vi "Telescope Update Status.vi"(8 "error in":errorcluster, 10 "Telescope Status":T2, 11 "HK Channel in":refnum<class "HK Table.lvclass">) -> (0 "error out":errorcluster, 2 "alarms":T1[](array[typedef]), 3 "HK Channel out":refnum<class "HK Table.lvclass">)   [LabVIEW 2021, in "Telescope.lvclass"]
uses:
  Telescope.lvclass
  Telescope cluster Status.ctl
  typedefs/CC cluster RA and DEC.ctl
  Telescope enum Status.ctl
  hk-channel-class/HK Table/HK Table.lvclass
  hk-channel-class/HK Alarms/HK Alarm enum Status.ctl
  hk-channel-class/HK Item/HK Item.lvclass
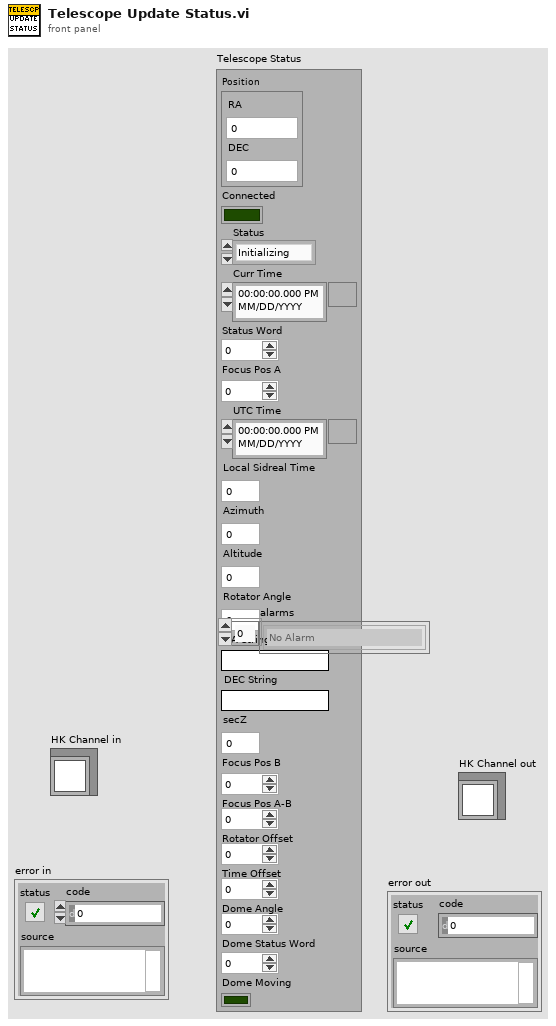
[diagram p1: front panel]
types:
  T1 = typedef "HK Item.lvclass/HK Alarm enum Status.ctl" = enum16{"No Alarm", "Red Low", "Red High", "Yellow Low", "Yellow High"}
  T2 = typedef "Telescope.lvclass/Telescope cluster Status.ctl" = cluster{"Position":T3, "Connected":bool, "Status":T4, "Curr Time":timestamp, "Status Word":u32, "Focus Pos A":dbl, "UTC Time":timestamp, "Local Sidreal Time":dbl, "Azimuth":dbl, "Altitude":dbl, "Rotator Angle":dbl, "RA String":string, "DEC String":string, "secZ":dbl, "Focus Pos B":dbl, "Focus Pos A-B":dbl, "Rotator Offset":dbl, "Time Offset":dbl, "Dome Angle":dbl, "Dome Status Word":u32, "Dome Moving":bool}
  T3 = typedef "CC cluster RA and DEC.ctl" = cluster{"RA":dbl, "DEC":dbl}
  T4 = typedef "Telescope.lvclass/Telescope enum Status.ctl" = enum16{"Initializing", "Ready", "Moving", "Focusing", "Error"}
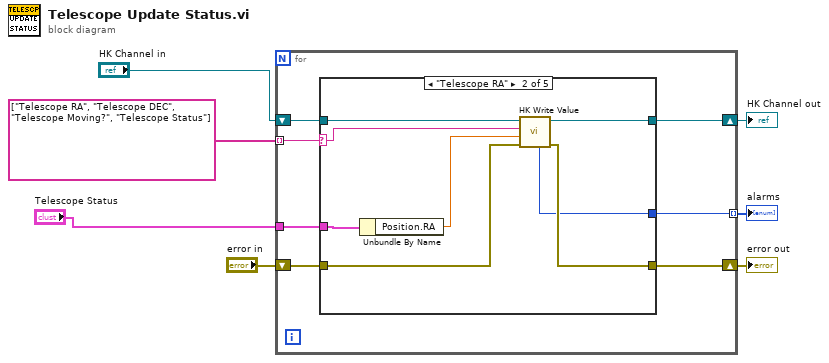
[diagram p0: block diagram]
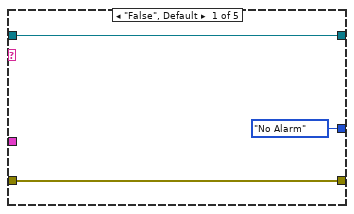
[diagram p2: hidden frame]
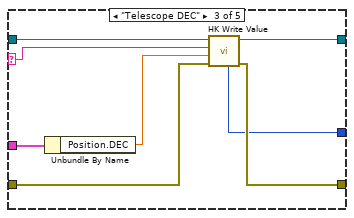
[diagram p3: hidden frame]
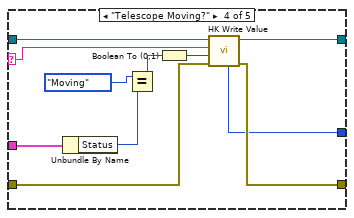
[diagram p4: hidden frame]
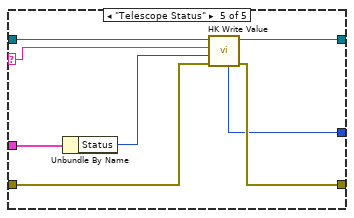
[diagram p5: hidden frame]
diagram:
  n1 = for {
    tunnel: string[] ["Telescope RA", "Telescope DEC", "Telescope Moving?", "Telescope Status"] -> [w14] mode=indexing
    shift-right: [w13] -> w2
    shift-left: "HK Channel in" -> [w12]
    shift-right: [w10] -> w4
    shift-left: "error in" -> [w11]
    tunnel: "Telescope Status" -> [w9]
    tunnel: [w8] -> w1 mode=indexing
    n2 = case shown="\"Telescope RA\"" w14 {
      selector: w14 -> [_ w23 w31 w42 w50]
      tunnel: [w17 w25 w33 w44 w52] -> w13
      tunnel: w12 -> [w17 w24 w32 w43 w51]
      tunnel: w11 -> [w16 w22 w30 w41 w49]
      tunnel: [w16 w21 w29 w40 w48] -> w10
      tunnel: w9 -> [_ w20 w28 w39 w47]
      tunnel: [HK_Alarm_enum_Status."No Alarm" ("Alarm Status") w18 w26 w34 w45] -> w8
      frame "False", Default {
      }
      frame "Telescope RA" {
        n3 = Unbundle By Name(w20) -> ("Position.RA"=w19:dbl)
        n4 = call-dynamic "HK Write Value.vi"("error in (no error)"=w22, "Value"=w19, "Channel Name"=w23, "HK Channel in"=w24) -> ("error out"=w21:errorcluster, "HK Channel out"=w25:refnum<class "HK Table.lvclass">, "Alarm Status"=w18:T1)  [unwired: 3 in, 2 out]
      }
      frame "Telescope DEC" {
        n5 = Unbundle By Name(w28) -> ("Position.DEC"=w27:dbl)
        n6 = call-dynamic "HK Write Value.vi"("error in (no error)"=w30, "Value"=w27, "Channel Name"=w31, "HK Channel in"=w32) -> ("error out"=w29:errorcluster, "HK Channel out"=w33:refnum<class "HK Table.lvclass">, "Alarm Status"=w26:T1)  [unwired: 3 in, 2 out]
      }
      frame "Telescope Moving?" {
        n7 = Unbundle By Name(w39) -> ("Status"=w38:T4)
        n8 = Equal?(x=Telescope_enum_Status."Moving" ("Status"), y=w38) -> (x = y?=w37:bool)
        n9 = Boolean To (0,1)(Boolean=w37) -> (0, 1=w35:i16)
        n10 = call-dynamic "HK Write Value.vi"("error in (no error)"=w41, "Value"=w35, "Channel Name"=w42, "HK Channel in"=w43) -> ("error out"=w40:errorcluster, "HK Channel out"=w44:refnum<class "HK Table.lvclass">, "Alarm Status"=w34:T1)  [unwired: 3 in, 2 out]
      }
      frame "Telescope Status" {
        n11 = Unbundle By Name(w47) -> ("Status"=w46:T4)
        n12 = call-dynamic "HK Write Value.vi"("error in (no error)"=w49, "Value"=w46, "Channel Name"=w50, "HK Channel in"=w51) -> ("error out"=w48:errorcluster, "HK Channel out"=w52:refnum<class "HK Table.lvclass">, "Alarm Status"=w45:T1)  [unwired: 3 in, 2 out]
      }
    }
  }
  "error out" <- w4
  "HK Channel out" <- w2
  "alarms" <- w1
